vi "Cleanup.vi"(8 "error in (no error)":errorcluster, 11 "Tread in":refnum<class "Tread.lvclass">) -> (0 "error out":errorcluster)   [LabVIEW 2020, in "Tread.lvclass"]
uses:
  Tread.lvclass
  Tread.lvclass/Tread.ctl
  nmea/nmea/VISA GPS/VISA GPS.lvclass
  bno055/BNO055/BNO055/BNO055.lvclass
  <vilib>/MakerHub/LINX/LMH-LINX.lvlib
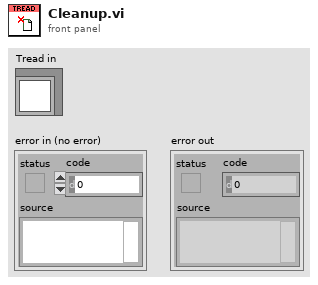
[diagram p1: front panel]
types:
  T1 = typedef "LMH-LINX.lvlib/LINX Ref.ctl" = cluster{"IO":T2, "Interface":T3, "LINX Device Config":T4}
  T2 = typedef "LMH-LINX.lvlib/Platform.ctl" = enum16{"Remote", "Local"}
  T3 = typedef "LMH-LINX.lvlib/Interface.ctl" = enum16{"Serial", "TCP"}
  T4 = typedef "LMH-LINX.lvlib/Device.lvlib/LINX Device Config.ctl" = cluster{"Interface":T3, "COM Port":refnum<visa-resource-name>, "TCP Configuration":T5, "Device Family":u8, "Device ID":u8, "Device Name":string, "TCP Ref":refnum<k5>, "Channels":T6}
  T5 = typedef "LMH-LINX.lvlib/Device.lvlib/TCP Config.ctl" = cluster{"IP Address":string, "Port":u16}
  T6 = typedef "LMH-LINX.lvlib/Channels.ctl" = cluster{"DI":u8[], "DO":u8[], "AI":u8[], "AO":u8[], "PWM":u8[], "QE":u8[], "UART":u8[], "I2C 2":u8[], "SPI":u8[], "CAN":u8[], "Servo":u8[], "AI Ref (V)":dbl, "AI Resolution (Bits)":u8, "AO Ref (V)":dbl, "AO Resolution (Bits)":u8}
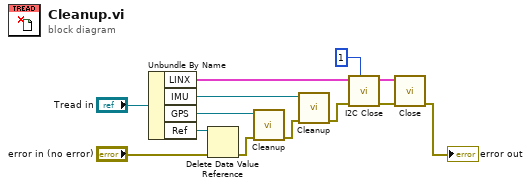
[diagram p0: block diagram]
diagram:
  n1 = Unbundle By Name("Tread in") -> ("LINX"=w7:T1, "IMU"=w9:refnum<class "BNO055.lvclass">, "GPS"=w11:refnum<class "VISA GPS.lvclass">, "Ref"=w12:refnum<data-value>)
  n2 = Delete Data Value Reference(data value reference=w12, error in="error in (no error)") -> (error out=w10:errorcluster)  [unwired: 1 out]
  n3 = call "Cleanup.vi"("error in (no error)"=w10, "VISA GPS in"=w11) -> ("error out"=w8:errorcluster)  [unwired: 9 in]
  n4 = call "Cleanup.vi"("error in (no error)"=w8, "BNO055 in"=w9) -> ("error out"=w6:errorcluster)  [unwired: 8 in, 1 out]
  n5 = call <vilib>:"I2C Close.vi"("I2C Channel (0)"=u8 1, "Error In"=w6, "LINX Resource"=w7) -> ("Error Out"=w4:errorcluster, "LINX Resource"=w3:T1)  [unwired: 7 in]
  n6 = call <vilib>:"Close.vi"("Error In"=w4, "LINX Resource"=w3) -> ("Error Out"=→"error out":errorcluster)  [unwired: 9 in]
